vi "WaitForREPL.vi"(8 "error in (no error)":errorcluster, 11 "Server":path) -> (0 "error out":errorcluster, 2 "REPL":string)   [LabVIEW 2020]
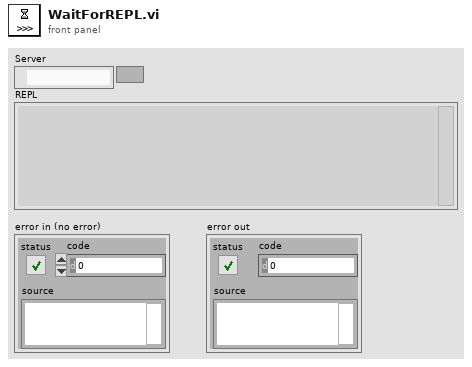
[diagram p1: front panel]
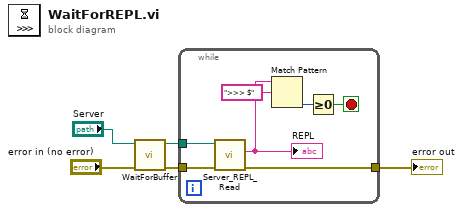
[diagram p0: block diagram]
diagram:
  n1 = call "WaitForBuffer.vi"("error in (no error)"="error in (no error)", "Server"="Server") -> ("error out"=w1:errorcluster)  [unwired: 8 in, 1 out]
  n2 = while {
    tunnel: w1 -> [w11]
    tunnel: "Server" -> [w10]
    tunnel: [w7] -> w4
    stop <- w8 stop-if-true
    n3 = call "Server_REPL_Read.vi"("error in (no error)"=w11, "Server"=w10) -> ("error out"=w7:errorcluster, "REPL"=w6:string)  [unwired: 7 in, 1 out]
    "REPL" <- w6
    n4 = Match Pattern(string=w6, regular expression=">>> $") -> (offset past match=w9:i32)  [unwired: 1 in, 3 out]
    n5 = Greater Or Equal To 0?(x=w9) -> (x >= 0?=w8:bool)
  }
  "error out" <- w4
